vi "E517_ErrorCheck.vi"(0 "Identification":string, 1 "Conn. Axes":string[](array[string]), 2 "Position":dbl[](array[numeric]) format="%.6f", 7 "error out 2":errorcluster) -> (13 "error IO":errorcluster)   [LabVIEW 2013]
uses:
  Variables/GlobalGetPhysikalInstrumentsOnOff.vi
  Variables/ScannerMirrorStatus.vi
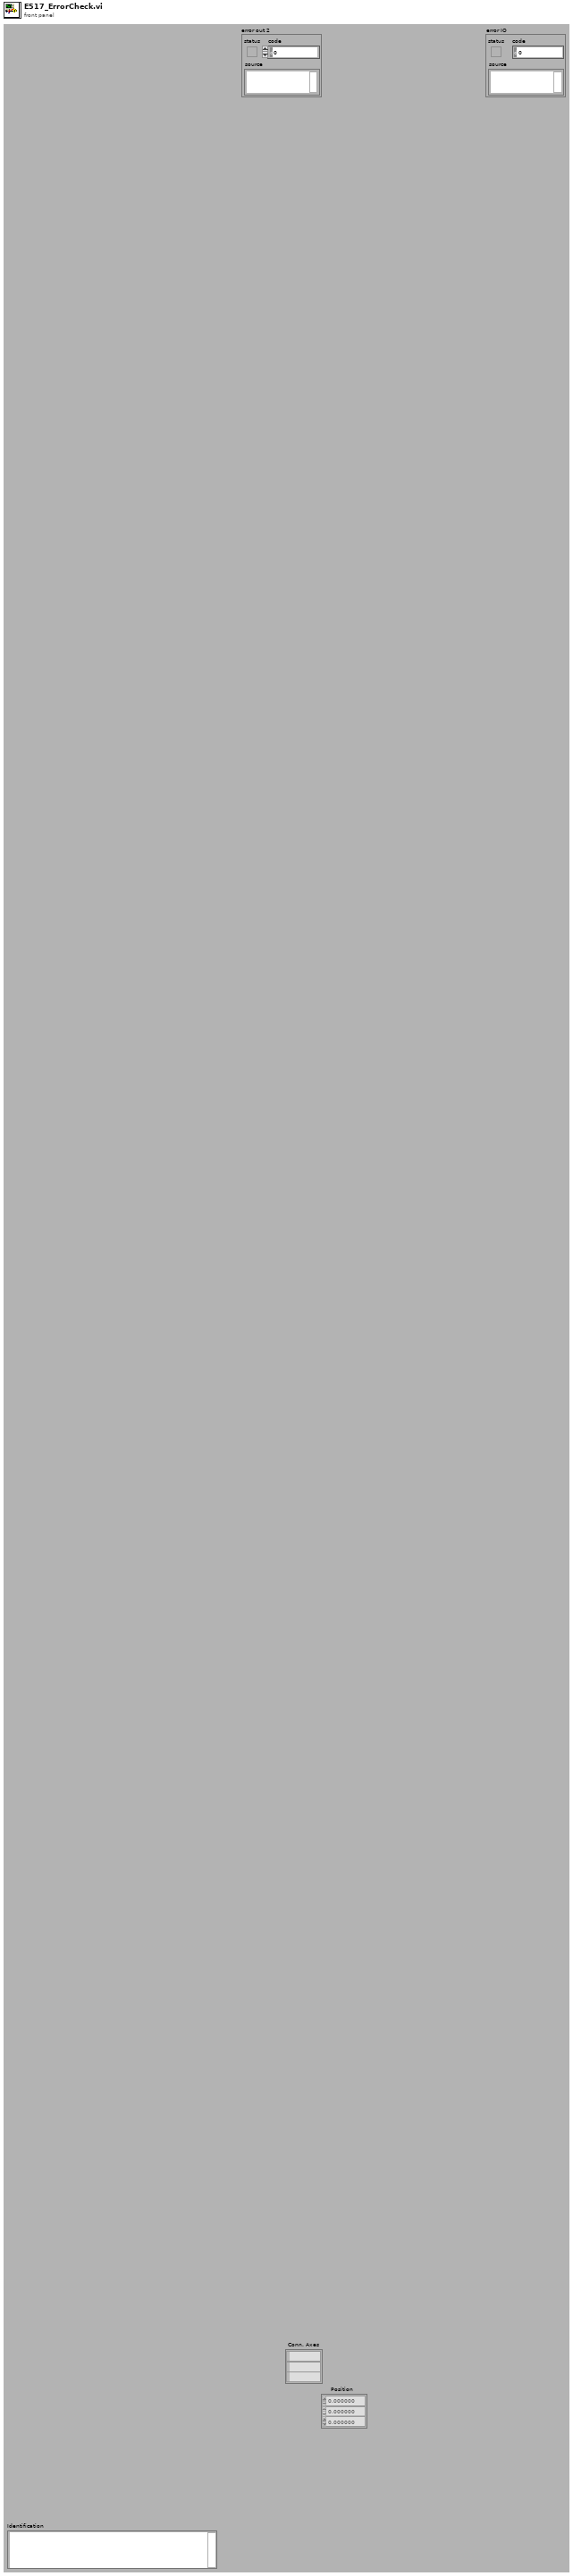
[diagram p1: front panel]
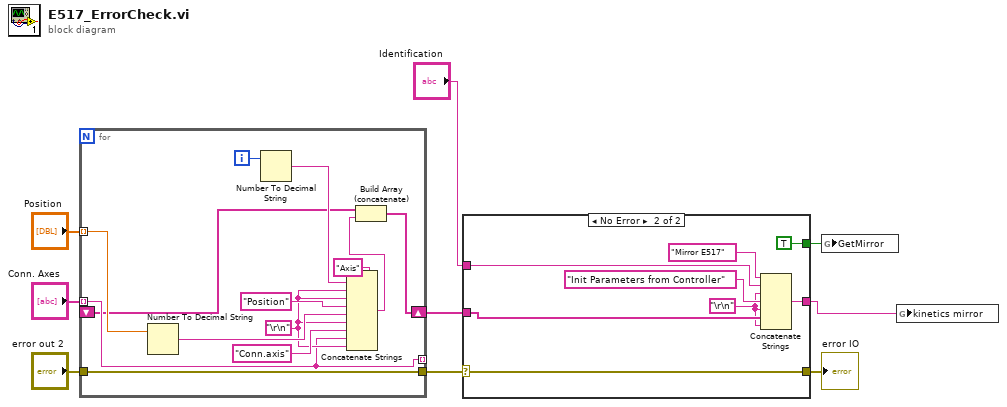
[diagram p0: block diagram]
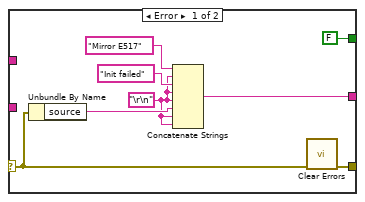
[diagram p2: hidden frame]
diagram:
  n1 = for {
    tunnel: "error out 2" -> [w19]
    tunnel: [w19] -> w5
    tunnel: "Position" -> [w17] mode=indexing
    tunnel: [w13] -> _ mode=indexing
    tunnel: "Conn. Axes" -> [w13] mode=indexing
    shift-right: [w11] -> w4
    shift-left: _ -> [w12]
    i -> [w22]
    w14 = "\r\n"
    n2 = Number To Decimal String(number=w17) -> (decimal integer string=w16:string)  [unwired: 1 in]
    n3 = Number To Decimal String(number=w22) -> (decimal integer string=w21:string)  [unwired: 1 in]
    n4 = Concatenate Strings("Axis", w21, w14, w14, "Position" ("string"), w16, w14, "Conn.axis" ("string"), w13, w14) -> (w10:string)
    n5 = Build Array (concatenate)(w12, w10) -> (w11:string[])
  }
  n6 = case shown="No Error" w5 {
    selector: w5 -> [w24 w36]
    tunnel: [w26 w36] -> w9
    tunnel: [w25 w37] -> w1
    tunnel: [FALSE ("Value") TRUE ("Value")] -> w8
    tunnel: "Identification" -> [_ w33]
    tunnel: w4 -> [_ w32]
    frame Error {
      w28 = "\r\n"
      n7 = Unbundle By Name(w24) -> ("source"=w29:string)
      n8 = Concatenate Strings("Mirror E517" ("string"), w28, "Init failed" ("string"), w28, w28, w29, w28, w28) -> (w25:string)
      n9 = call <vilib>:"Clear Errors.vi"("error in (no error)"=w24) -> ("error out"=w26:errorcluster)  [unwired: 6 in]
    }
    frame No Error {
      w31 = "\r\n"
      n10 = Concatenate Strings("Mirror E517" ("string"), w33, w31, "Init Parameters from Controller" ("string"), w31, w32, w31) -> (w37:string)
    }
  }
  "error IO" <- w9
  n11 = global write "GlobalGetPhysikalInstrumentsOnOff.vi" "GetMirror"(w8) -> ()
  n12 = global write "ScannerMirrorStatus.vi" "kinetics mirror"(w1) -> ()
